vi "Load_from_Project.vi"(8 "error in (no error)":errorcluster, 9 "index":string, 10 "buildObject":T1, 11 "IB_Source_File in":refnum<class "IB_Source_File.lvclass">) -> (0 "error out":errorcluster, 1 "index out":string, 2 "buildObject out":T1, 3 "IB_Source_File out":refnum<class "IB_Source_File.lvclass">)   [LabVIEW 2020, in "IB_Source_File.lvclass"]
uses:
  <vilib>/AppBuilder/IB_Classes/Source/File/IB_Source_File.lvclass
  <vilib>/AppBuilder/IB_Classes/Source/File/IB_Source_File.lvclass/IB_Source_File.ctl
  <vilib>/AppBuilder/IB_RW_Project/IB_RW_Project_PropBag_Action.ctl
  <vilib>/AppBuilder/IB_Classes/Shortcut/IB_Shortcut.lvclass
  <vilib>/AppBuilder/IB_Classes/Source/IB_Source.lvclass
  <resource>/Framework/Providers/API/ItemRef.ctl
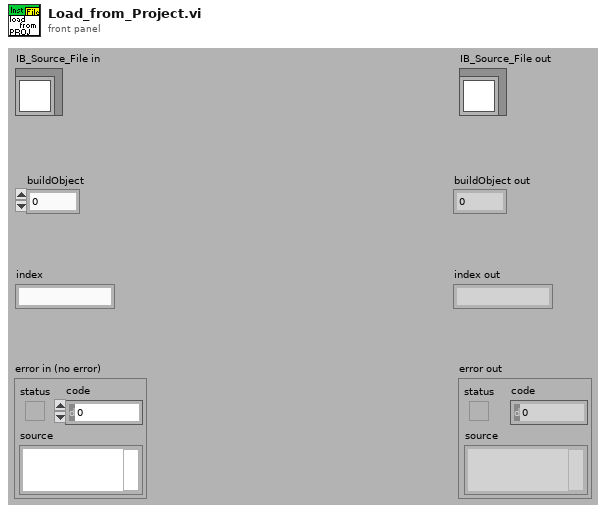
[diagram p1: front panel]
types:
  T1 = typedef "ItemRef.ctl" = u64
  T2 = typedef "IB_RW_Project_PropBag_Action.ctl" = enum16{"read", "write", "clear", "readPrevious", "writePrevious", "clearPrevious"}
  T3 = typedef "IB_RW_Project_Source_File_Data.ctl" = cluster{"attributes":i16, "RegCOM":bool, "unlock":bool, "runEXE":bool, "cmdArg":string, "EXE_uninstall":bool, "CmdArg_uninstsall":string}
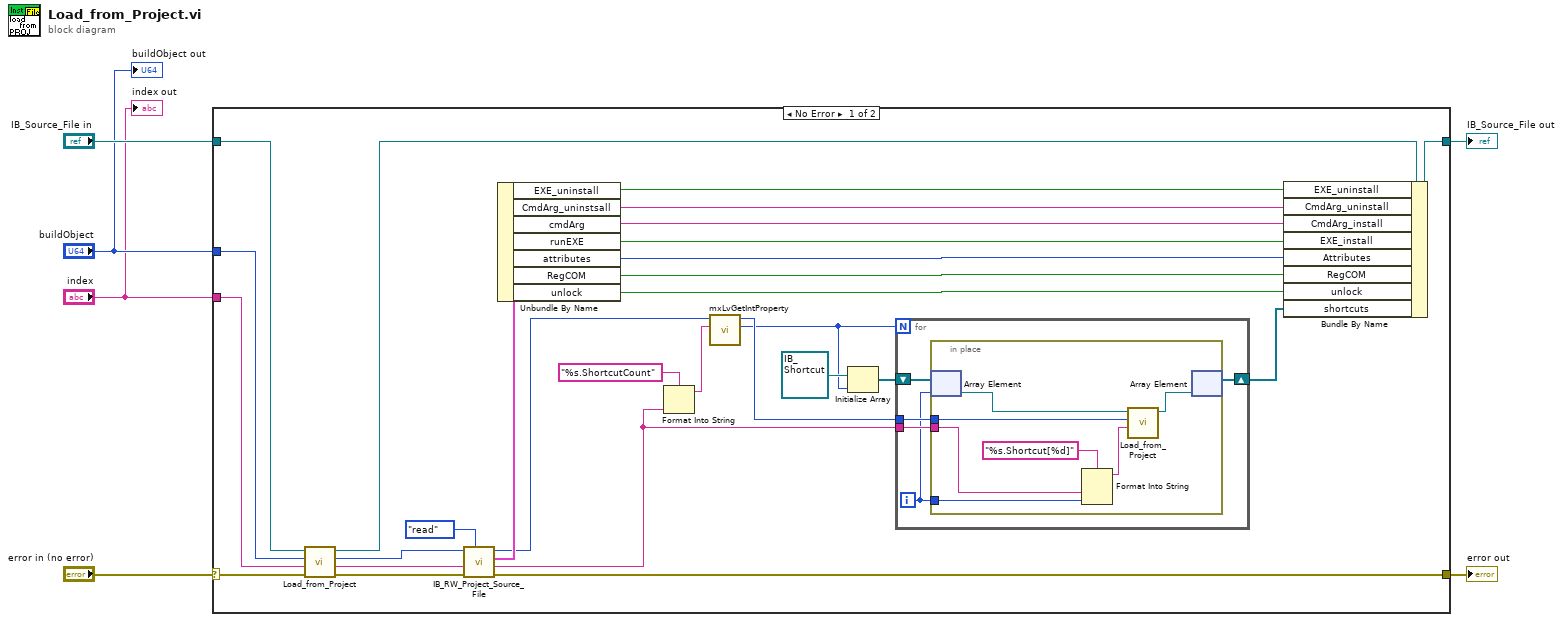
[diagram p0: block diagram]
diagram:
  n1 = case shown="No Error" "error in (no error)" {
    selector: "error in (no error)" -> [w32 w48]
    tunnel: [w29 w48] -> w6
    tunnel: [w23 w47] -> w5
    tunnel: "index" -> [w34 _]
    tunnel: "buildObject" -> [w28 _]
    tunnel: "IB_Source_File in" -> [w33 w47]
    frame No Error {
      n2 = call-parent <vilib>:"Load_from_Project.vi"("error in (no error)"=w32, "index in"=w34, "buildObject"=w28, "IB_Source in"=w33) -> ("error out"=w30:errorcluster, "index out"=w26:string, "buildObject out"=w27:T1, "IB_Source out"=w24:refnum<class "IB_Source_File.lvclass">)  [unwired: 4 out]
      n3 = call <vilib>:"IB_RW_Project_Source_File.vi"("action"=IB_RW_Project_PropBag_Action."read", "error in (no error)"=w30, "index in"=w26, "buildObject"=w27) -> ("error out"=w29:errorcluster, "index out"=w16:string, "file out"=w25:T3, "buildObject out"=w19:T1)  [unwired: 1 in, 3 out]
      n4 = Unbundle By Name(w25) -> ("EXE_uninstall"=w8:bool, "CmdArg_uninstsall"=w7:string, "cmdArg"=w10:string, "runEXE"=w9:bool, "attributes"=w22:i16, "RegCOM"=w21:bool, "unlock"=w20:bool)
      n5 = Format Into String(format string="%s.ShortcutCount", w16) -> (resulting string=w17:string)  [unwired: 2 in, 1 out]
      n6 = call <resource>:"mxLvGetIntProperty.vi"("Tag"=w17, "Item"=w19) -> ("Value"=w12:i32, "Item"=w15:T1)  [unwired: 1 in, 7 out]
      n7 = Initialize Array(refnum<class "IB_Shortcut.lvclass"> refnum ("IB_Shortcut.lvclass"), w12) -> (w13:refnum<class "IB_Shortcut.lvclass">[])
      n8 = for {
        N: w12 -> [_]
        tunnel: w16 -> [w39]
        tunnel: w15 -> [w38]
        shift-right: [w36] -> w11
        shift-left: w13 -> [w37]
        i -> [w35]
        n9 = in-place {
          in-place-border: w39 -> [w41]
          in-place-border: w38 -> [w46]
          in-place-border: w35 -> [w42]
          n10 = in-place-array #1(w37, w35) -> (w45:refnum<class "IB_Shortcut.lvclass">)
          n11 = Format Into String(format string="%s.Shortcut[%d]", w41, w42) -> (resulting string=w40:string)  [unwired: 2 in, 1 out]
          n12 = call <vilib>:"Load_from_Project.vi"("index"=w40, "buildObject"=w46, "IB_Shortcut in"=w45) -> ("IB_Shortcut out"=w44:refnum<class "IB_Shortcut.lvclass">)  [unwired: 1 in, 7 out]
          n13 = in-place-array #1(w44) -> (w36:refnum<class "IB_Shortcut.lvclass">[])  [unwired: 1 out]
        }
      }
      n14 = Bundle By Name(cluster=w24, "EXE_uninstall"=w8, "CmdArg_uninstall"=w7, "CmdArg_install"=w10, "EXE_install"=w9, "Attributes"=w22, "RegCOM"=w21, "unlock"=w20, "shortcuts"=w11) -> (w23:refnum<class "IB_Source_File.lvclass">)
    }
    frame Error {
    }
  }
  "error out" <- w6
  "IB_Source_File out" <- w5
  "buildObject out" <- "buildObject"
  "index out" <- "index"
